vi "ReadFilterParam (SubVI).vi"(8 "error in (no error)":errorcluster, 10 "section":string="LPF_7MHz5", 11 "Refnum in":T1) -> (0 "error out":errorcluster, 1 "BodePlot":cluster{"Frq":dbl[], "Kt":dbl[]}, 3 "Refnum out":T1)   [LabVIEW 2017]
uses:
  <vilib>/Utility/config.llb/Config Data RefNum.ctl
  <vilib>/Utility/config.llb/Read Key (Double).vi
  <vilib>/Utility/config.llb/NI_LVConfig.lvlib
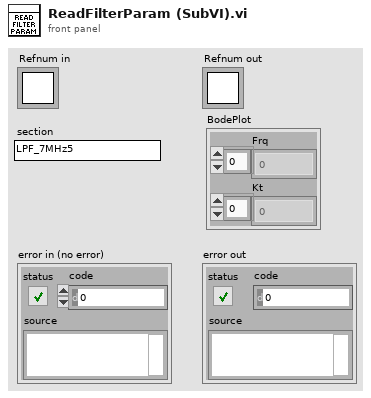
[diagram p1: front panel]
types:
  T1 = typedef "NI_LVConfig.lvlib/Config Data RefNum.ctl" = refnum<k1>
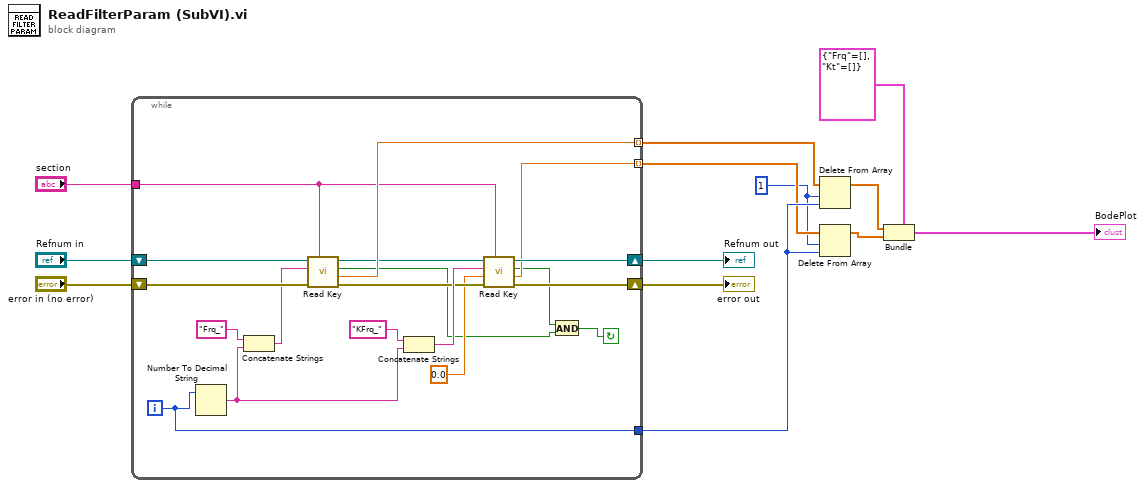
[diagram p0: block diagram]
diagram:
  w5 = 1 ("length")
  n1 = while {
    shift-right: [w22] -> w11
    shift-left: "Refnum in" -> [w32]
    shift-right: [w21] -> w12
    shift-left: "error in (no error)" -> [w31]
    tunnel: [w30] -> w8 mode=indexing
    tunnel: [w20] -> w6 mode=indexing
    tunnel: "section" -> [w19]
    tunnel: [w14] -> w7
    i -> [w14]
    stop <- w15 continue-if-true
    n2 = Number To Decimal String(number=w14) -> (decimal integer string=w26:string)  [unwired: 1 in]
    n3 = Concatenate Strings("Frq_" ("key"), w26) -> (w28:string)
    n4 = call-poly <vilib>:"Read Key.vi"("section"=w19, "error in (no error)"=w31, "key"=w28, "refnum"=w32) -> ("error out"=w23:errorcluster, "value"=w30:dbl, "found?"=w16:bool, "refnum out"=w25:T1)  [unwired: 2 in, 2 out]
    n5 = Concatenate Strings("KFrq_" ("key"), w26) -> (w24:string)
    n6 = call-poly <vilib>:"Read Key.vi"("section"=w19, "error in (no error)"=w23, "default value"=0.0, "key"=w24, "refnum"=w25) -> ("error out"=w21:errorcluster, "value"=w20:dbl, "found?"=w17:bool, "refnum out"=w22:T1)  [unwired: 1 in, 2 out]
    n7 = And(x=w17, y=w16) -> (x .and. y?=w15:bool)
  }
  "error out" <- w12
  "Refnum out" <- w11
  n8 = Delete From Array(array=w8, length=w5, index=w7) -> (array with subset deleted=w4:dbl[])  [unwired: 1 out]
  n9 = Delete From Array(array=w6, length=w5, index=w7) -> (array with subset deleted=w1:dbl[])  [unwired: 1 out]
  n10 = Bundle(cluster=cluster{"Frq":dbl[], "Kt":dbl[]} {"Frq"=[], "Kt"=[]}, "Frq"=w4, "Kt"=w1) -> (→"BodePlot":cluster{"Frq":dbl[], "Kt":dbl[]})
